vi "Untitled 1.vi"() -> ()   [LabVIEW 2013]
panel:
  out "time diff 2":u32
  out "recieved":i32
  in  "y":bool
  out "data out":string
  out "error out":errorcluster
  out "time diff":u32
  in  "stop":bool
  out "remote address":string
  in  "Port number":dbl=1.0 min=1.0 max=49150.0 step=1.0
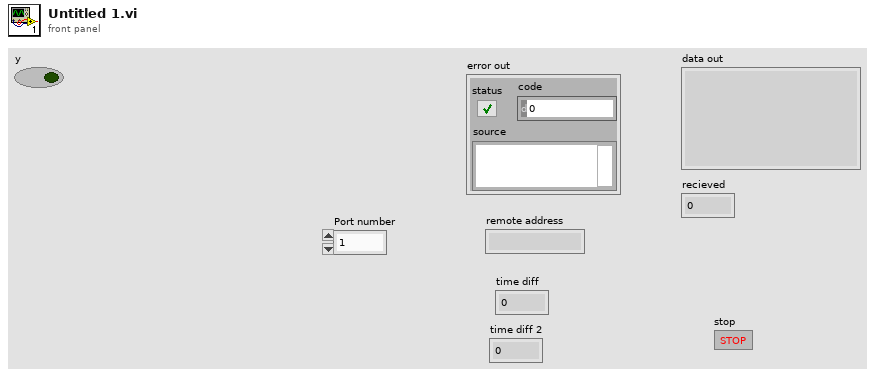
[diagram p1: front panel]
types:
  T1 = enum16{"Standard", "Buffered", "CRLF", "Immediate"}
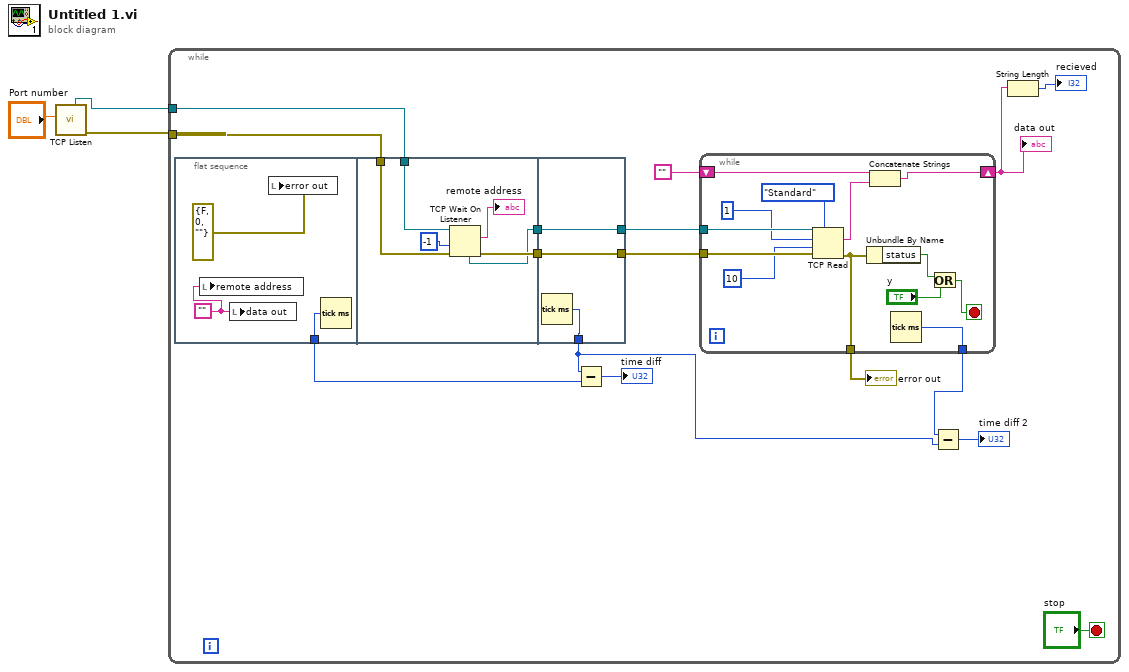
[diagram p0: block diagram]
diagram:
  n1 = call <vilib>:"TCP Listen.vi"("port"="Port number") -> ("error out"=w2:errorcluster, "listener ID"=w1:refnum<k5>)  [unwired: 6 in, 3 out]
  n2 = while {
    tunnel: w1 -> [w16]
    tunnel: w2 -> [w15]
    stop <- "stop" stop-if-true
    n3 = flat-sequence {
      tunnel: [w35] -> w18
      tunnel: w16 -> [w40]
      tunnel: w15 -> [w39]
      tunnel: [w36] -> w14
      tunnel: [w37] -> w13
      tunnel: [w44] -> w4
      tunnel: [w43] -> w11
      tunnel: w14 -> [w43]
      tunnel: [w42] -> w12
      tunnel: w13 -> [w42]
      frame #0 {
        w34 = ""
        n4 = local write "remote address"(w34) -> ()
        n5 = local write "data out"(w34) -> ()
        n6 = local write "error out"(errorcluster {"status"=FALSE, "code"=0, "source"=""} ("error out")) -> ()
        n7 = Tick Count (ms)() -> (millisecond timer value=w35:u32)
      }
      frame #1 {
        n8 = TCP Wait On Listener(8:w39, 9:-1 ("timeout ms (wait forever: -1)"), 11:w40) -> (0:w37:errorcluster, 2:→"remote address":string, 4:w36:refnum<k5>)  [unwired: 1 in, 2 out]
      }
      frame #2 {
        n9 = Tick Count (ms)() -> (millisecond timer value=w44:u32)
      }
    }
    n10 = Subtract(x=w4, y=w18) -> (x-y=→"time diff":u32)
    n11 = while {
      tunnel: w12 -> [w32]
      tunnel: w11 -> [w31]
      tunnel: [w28] -> w10
      shift-right: [w24] -> w8
      shift-left: "" -> [w23]
      tunnel: [w20] -> w5
      stop <- w26 stop-if-true
      n12 = TCP Read(connection ID=w31, bytes to read=1, error in (no error)=w32, 7:T1."Standard" ("mode (standard)"), 9:10 ("timeout ms (25000)")) -> (data out=w22:string, error out=w28:errorcluster)  [unwired: 1 out]
      n13 = Unbundle By Name(w28) -> ("status"=w27:bool)
      n14 = Concatenate Strings(w23, w22) -> (w24:string)
      n15 = Tick Count (ms)() -> (millisecond timer value=w20:u32)
      n16 = Or(x=w27, y="y") -> (x .or. y?=w26:bool)
    }
    "error out" <- w10
    "data out" <- w8
    n17 = Subtract(x=w5, y=w4) -> (x-y=→"time diff 2":u32)
    n18 = String Length(string=w8) -> (length=→"recieved":i32)
  }
